vi "Read_Logger.vi"(4 "Input String":string, 5 "Msg In":u8=255, 6 "aDATA":u8[](array[numeric])) -> (0 "Output String":string, 1 "End of Log":bool, 2 "Msg out":u8=255, 3 "Send_Msg":bool)   [LabVIEW 2010]
panel:
  in  "Type of message":bool
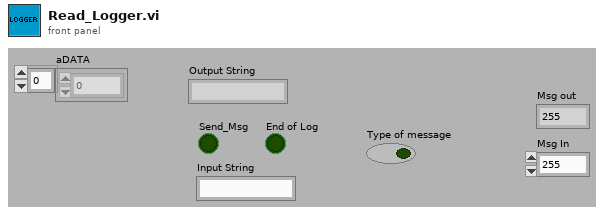
[diagram p1: front panel]
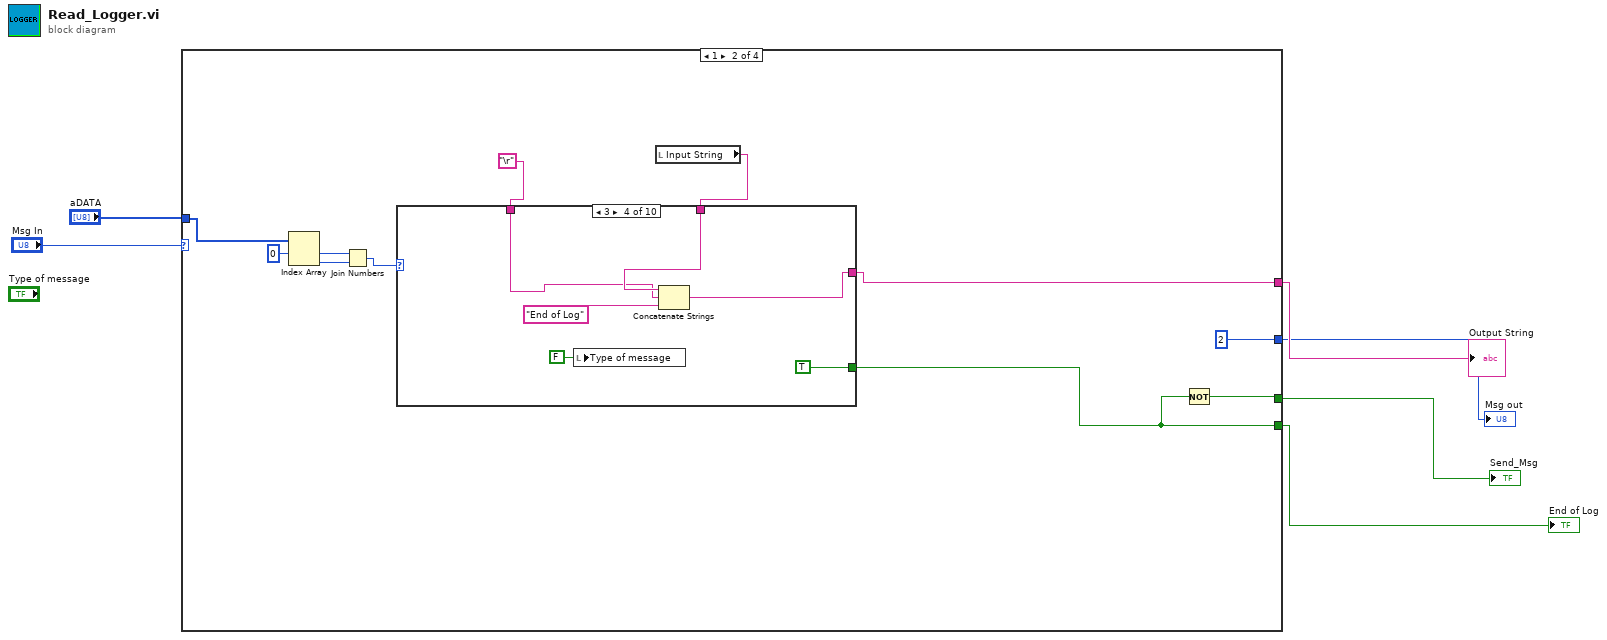
[diagram p0: block diagram]
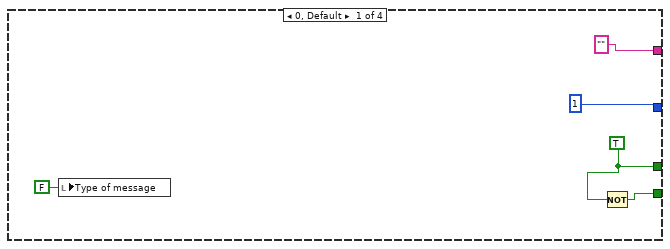
[diagram p2: hidden frame]
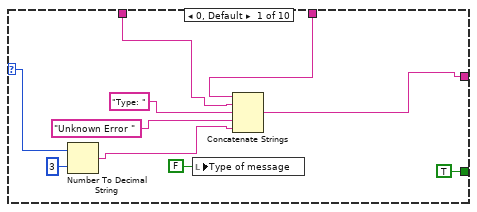
[diagram p3: hidden frame]
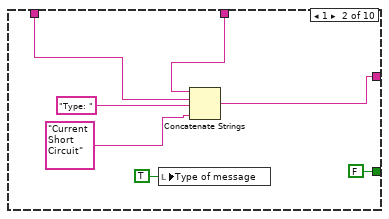
[diagram p4: hidden frame]
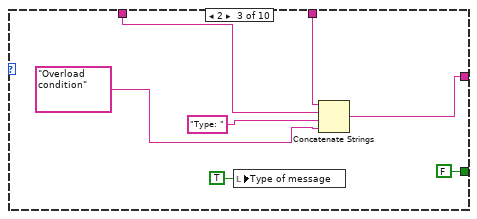
[diagram p5: hidden frame]
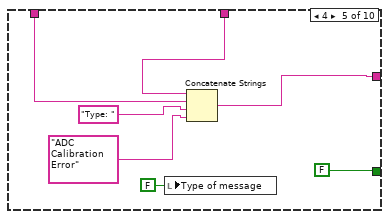
[diagram p6: hidden frame]
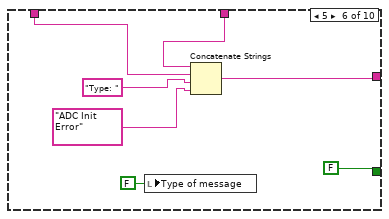
[diagram p7: hidden frame]
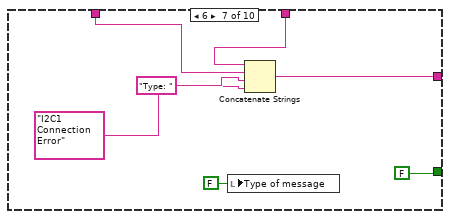
[diagram p8: hidden frame]
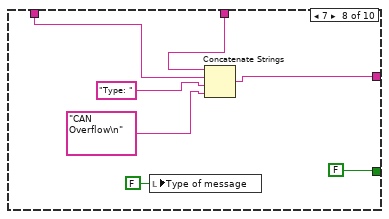
[diagram p9: hidden frame]
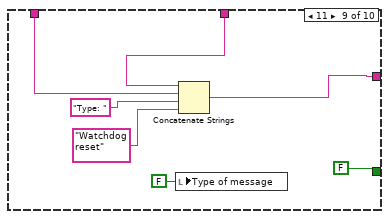
[diagram p10: hidden frame]
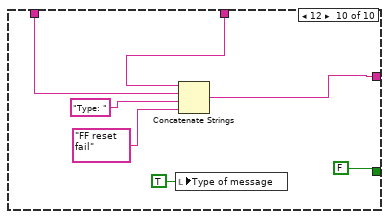
[diagram p11: hidden frame]
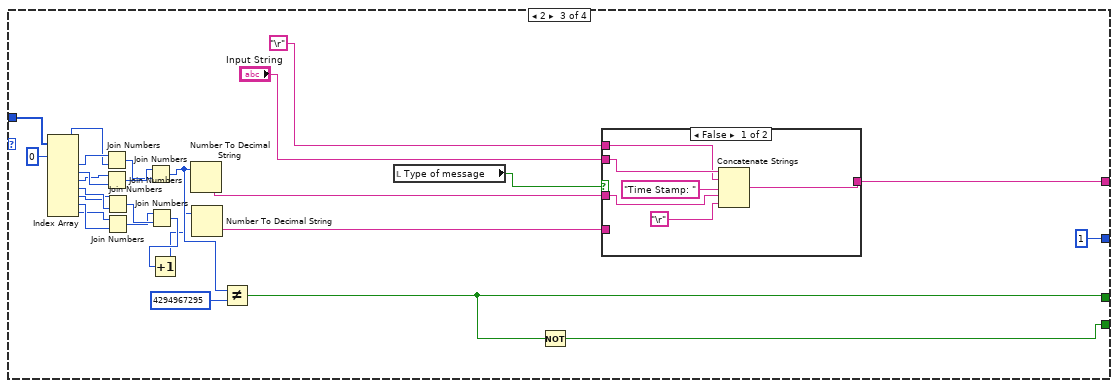
[diagram p12: hidden frame]
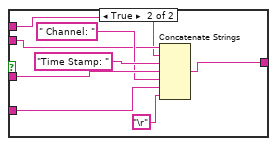
[diagram p13: hidden frame]
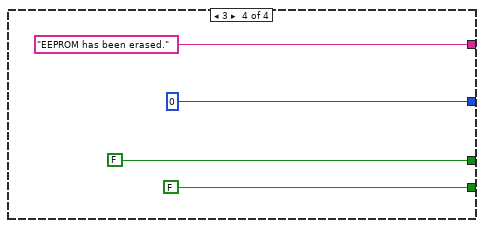
[diagram p14: hidden frame]
diagram:
  n1 = case shown="1" "Msg In" {
    tunnel: "aDATA" -> [_ w21 w121 _]
    tunnel: ["" w16 w111 "EEPROM has been erased."] -> w5
    tunnel: [u8 1 ("Type of msg in 2") u8 2 ("Type of msg in 2") u8 1 ("Type of msg in 2") u8 0 ("Type of msg in 2")] -> w3
    tunnel: [w8 w12 w97 FALSE ("Read_Log")] -> w2
    tunnel: [w9 w13 w96 FALSE ("End of log")] -> w1
    frame 0, Default {
      w8 = TRUE ("End of log")
      n2 = local write "Type of message"(FALSE ("Type of message")) -> ()
      n3 = Not(x=w8) -> (.not. x?=w9:bool)
    }
    frame 1 {
      n4 = Index Array(array=w21, index #1=0 ("index")) -> (element #1=w19:u8, element #2=w18:u8)  [unwired: 1 in]
      n5 = Join Numbers(hi=w18, lo=w19) -> ((hi.lo)=w17:u16)
      n6 = local read "Input String"() -> (w15:string)
      n7 = case shown="3" w17 {
        selector: w17 -> [w25 _ _ _ _ _ _ _ _ _]
        tunnel: [w29 w38 w44 w52 w56 w63 w70 w77 w84 w91] -> w16
        tunnel: w15 -> [w30 w37 w43 w49 w59 w64 w71 w78 w81 w88]
        tunnel: "\r" -> [w26 w33 w40 w48 w53 w60 w67 w74 w87 w94]
        tunnel: [TRUE ("Read_Log") FALSE ("Read_Log") FALSE ("Read_Log") TRUE ("Read_Log") FALSE ("Read_Log") FALSE ("Read_Log") FALSE ("Read_Log") FALSE ("Read_Log") FALSE ("Read_Log") FALSE ("Read_Log")] -> w13
        frame 0, Default {
          n8 = Number To Decimal String(number=w25, width (-)=i16 3) -> (decimal integer string=w24:string)
          n9 = local write "Type of message"(FALSE ("Type of message")) -> ()
          n10 = Concatenate Strings(w30, w26, "Type: " ("string"), "Unknown Error " ("string"), w24) -> (w29:string)
        }
        frame 1 {
          n11 = local write "Type of message"(TRUE ("Type of message")) -> ()
          n12 = Concatenate Strings(w37, w33, "Type: " ("string"), "Current Short Circuit" ("string")) -> (w38:string)
        }
        frame 2 {
          n13 = local write "Type of message"(TRUE ("Type of message")) -> ()
          n14 = Concatenate Strings(w43, w40, "Type: " ("string"), "Overload condition" ("string")) -> (w44:string)
        }
        frame 3 {
          n15 = local write "Type of message"(FALSE ("Type of message")) -> ()
          n16 = Concatenate Strings(w49, w48, "End of Log" ("string")) -> (w52:string)
        }
        frame 4 {
          n17 = local write "Type of message"(FALSE ("Type of message")) -> ()
          n18 = Concatenate Strings(w59, w53, "Type: " ("string"), "ADC Calibration Error" ("string")) -> (w56:string)
        }
        frame 5 {
          n19 = local write "Type of message"(FALSE ("Type of message")) -> ()
          n20 = Concatenate Strings(w64, w60, "Type: " ("string"), "ADC Init Error" ("string")) -> (w63:string)
        }
        frame 6 {
          n21 = local write "Type of message"(FALSE ("Type of message")) -> ()
          n22 = Concatenate Strings(w71, w67, "Type: " ("string"), "I2C1 Connection Error" ("string")) -> (w70:string)
        }
        frame 7 {
          n23 = local write "Type of message"(FALSE ("Type of message")) -> ()
          n24 = Concatenate Strings(w78, w74, "Type: " ("string"), "CAN Overflow\n" ("string")) -> (w77:string)
        }
        frame 11 {
          n25 = local write "Type of message"(FALSE ("Type of message")) -> ()
          n26 = Concatenate Strings(w81, w87, "Type: " ("string"), "Watchdog reset" ("string")) -> (w84:string)
        }
        frame 12 {
          n27 = local write "Type of message"(TRUE ("Type of message")) -> ()
          n28 = Concatenate Strings(w88, w94, "Type: " ("string"), "FF reset fail" ("string")) -> (w91:string)
        }
      }
      n29 = Not(x=w13) -> (.not. x?=w12:bool)
    }
    frame 2 {
      n30 = Index Array(array=w121, index #1=0 ("index")) -> (element #1=w106:u8, element #2=w107:u8, element #3=w105:u8, element #4=w104:u8, element #5=w101:u8, element #6=w100:u8, element #7=w103:u8, element #8=w102:u8)  [unwired: 7 in]
      n31 = Join Numbers(hi=w107, lo=w106) -> ((hi.lo)=w118:u16)
      n32 = Join Numbers(hi=w104, lo=w105) -> ((hi.lo)=w119:u16)
      n33 = Join Numbers(hi=w100, lo=w101) -> ((hi.lo)=w116:u16)
      n34 = Join Numbers(hi=w102, lo=w103) -> ((hi.lo)=w115:u16)
      n35 = Join Numbers(hi=w119, lo=w118) -> ((hi.lo)=w109:u32)
      n36 = Join Numbers(hi=w115, lo=w116) -> ((hi.lo)=w99:u32)
      n37 = Increment(x=w99) -> (x+1=w98:u32)
      n38 = Number To Decimal String(number=w109) -> (decimal integer string=w117:string)  [unwired: 1 in]
      n39 = Number To Decimal String(number=w98) -> (decimal integer string=w114:string)  [unwired: 1 in]
      n40 = Not Equal?(x=w109, y=u32 4294967295) -> (x != y?=w97:bool)
      n41 = local read "Type of message"() -> (w95:bool)
      n42 = Not(x=w97) -> (.not. x?=w96:bool)
      n43 = case shown="False" w95 {
        tunnel: w117 -> [w123 w134]
        tunnel: w114 -> [_ w132]
        tunnel: "Input String" -> [w127 w131]
        tunnel: "\r" -> [w126 w130]
        tunnel: [w125 w129] -> w111
        frame False {
          n44 = Concatenate Strings(w127, w126, "Time Stamp: " ("string"), w123, "\r") -> (w125:string)
        }
        frame True {
          n45 = Concatenate Strings(w131, w130, "Time Stamp: " ("string"), w134, " Channel: " ("string"), w132, "\r") -> (w129:string)
        }
      }
    }
    frame 3 {
    }
  }
  "Output String" <- w5
  "Msg out" <- w3
  "Send_Msg" <- w2
  "End of Log" <- w1
